vi "Example Callback - Coordinates Callback.vi"(4 "Coordinates":refnum<user-event>, 5 "Event Data":T1, 6 "Control Ref":refnum<k24>, 7 "Event Common Data":T2) -> ()   [LabVIEW 2013]
uses:
  C:/tf/play/labview/Tinkerforge.dll
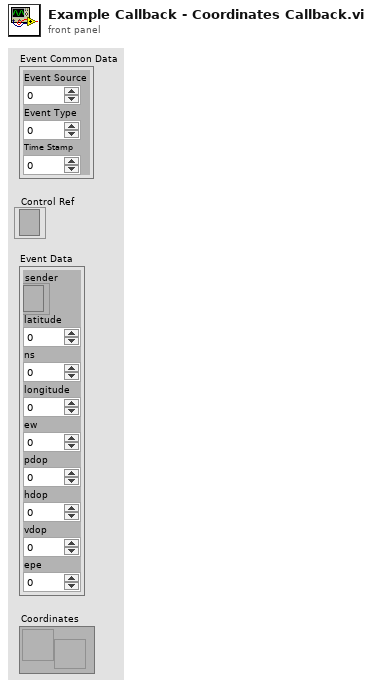
[diagram p1: front panel]
types:
  T1 = cluster{"sender":refnum<k24>, "latitude":i64, "ns":u16, "longitude":i64, "ew":u16, "pdop":i32, "hdop":i32, "vdop":i32, "epe":i32}
  T2 = cluster{"Event Source":i32, "Event Type":u32, "Time Stamp":u32}
  T3 = cluster{"latitude":i64, "ns":u16, "longitude":i64, "ew":u16, "pdop":i32, "hdop":i32, "vdop":i32, "epe":i32}
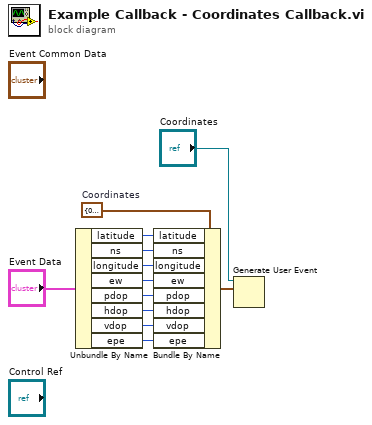
[diagram p0: block diagram]
diagram:
  w11 = T3 {"latitude"=0, "ns"=0, "longitude"=0, "ew"=0, "pdop"=0, "hdop"=0, "vdop"=0, "epe"=0}  # Coordinates
  n1 = Unbundle By Name("Event Data") -> ("latitude"=w8:i64, "ns"=w7:u16, "longitude"=w6:i64, "ew"=w5:u16, "pdop"=w4:i32, "hdop"=w3:i32, "vdop"=w2:i32, "epe"=w1:i32)
  n2 = Bundle By Name(cluster=w11, "latitude"=w8, "ns"=w7, "longitude"=w6, "ew"=w5, "pdop"=w4, "hdop"=w3, "vdop"=w2, "epe"=w1) -> (w10:T3)
  n3 = Generate User Event(user event="Coordinates", event data cluster=w10) -> ()  [unwired: 2 in, 2 out]
